vi "AB_850_860_Project_Source_Container.vi"(7 "action":T3, 8 "error in (no error)":errorcluster, 9 "index in":i32, 10 "dataSource in":T2, 11 "buildObject":T1) -> (0 "error out":errorcluster, 1 "index out":i32, 2 "dataSource out":T2, 3 "buildObject out":T1)   [LabVIEW 2020]
doc: "Reads and writes the data to the object property bag."
uses:
  <resource>/Framework/Providers/API/ItemRef.ctl
  <vilib>/AppBuilder/RW_Project/AB_RW_Project_PropBag_Action.ctl
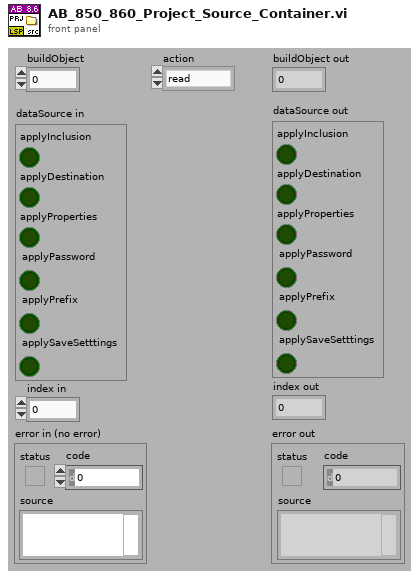
[diagram p1: front panel]
types:
  T1 = typedef "ItemRef.ctl" = u64
  T2 = cluster{"applyInclusion":bool, "applyDestination":bool, "applyProperties":bool, "applyPassword":bool, "applyPrefix":bool, "applySaveSetttings":bool}
  T3 = typedef "AB_RW_Project_PropBag_Action.ctl" = enum16{"read", "write", "clear", "readPrevious", "writePrevious", "clearPrevious"}
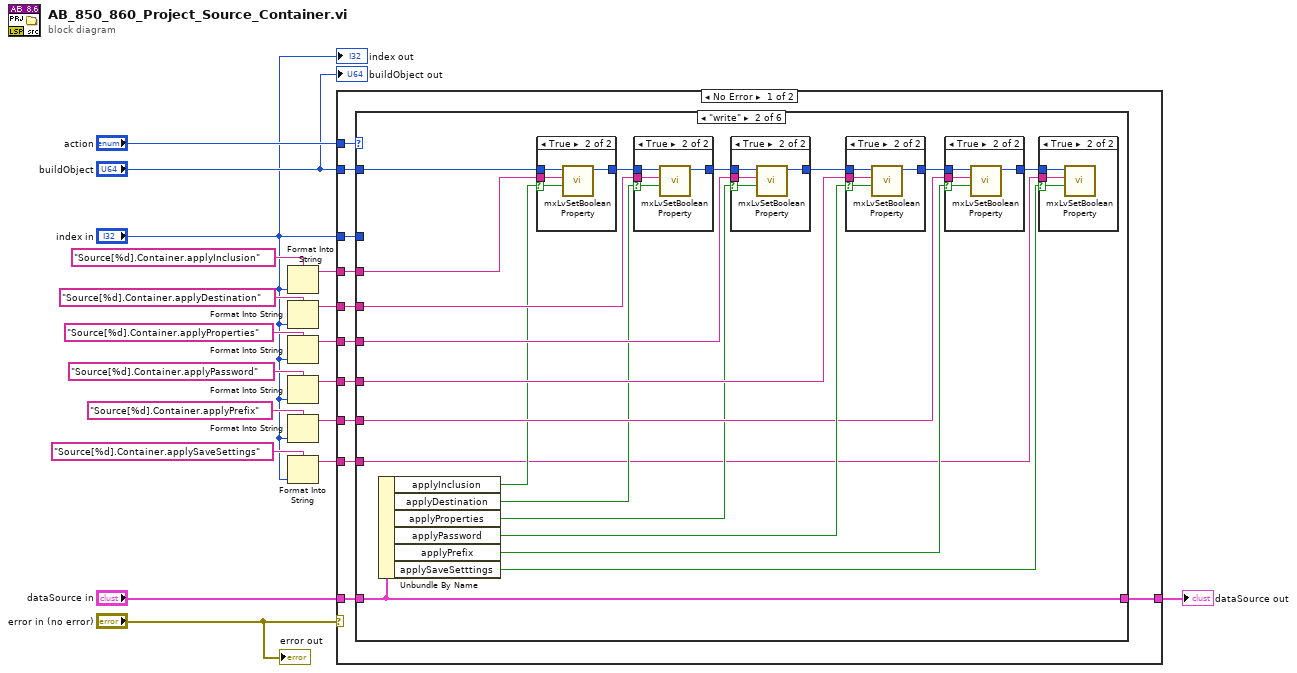
[diagram p0: block diagram]
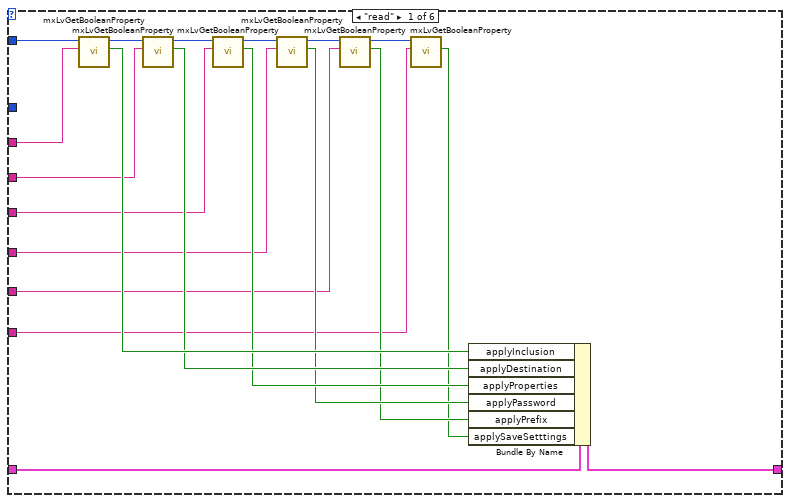
[diagram p2: hidden frame]
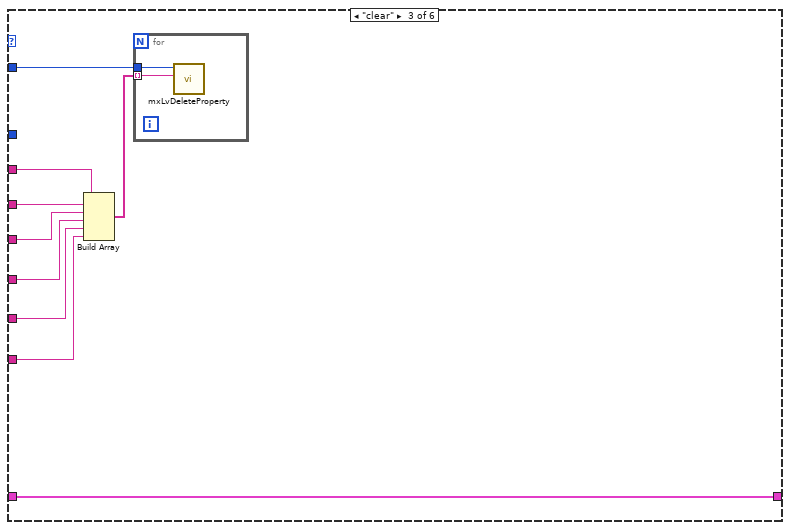
[diagram p9: hidden frame]
diagram:
  n1 = Format Into String(format string="Source[%d].Container.applyInclusion", "index in") -> (resulting string=w15:string)  [unwired: 2 in, 1 out]
  n2 = Format Into String(format string="Source[%d].Container.applyDestination", "index in") -> (resulting string=w12:string)  [unwired: 2 in, 1 out]
  n3 = Format Into String(format string="Source[%d].Container.applyProperties", "index in") -> (resulting string=w11:string)  [unwired: 2 in, 1 out]
  n4 = Format Into String(format string="Source[%d].Container.applyPassword", "index in") -> (resulting string=w6:string)  [unwired: 2 in, 1 out]
  n5 = Format Into String(format string="Source[%d].Container.applyPrefix", "index in") -> (resulting string=w4:string)  [unwired: 2 in, 1 out]
  n6 = Format Into String(format string="Source[%d].Container.applySaveSettings", "index in") -> (resulting string=w1:string)  [unwired: 2 in, 1 out]
  n7 = case shown="No Error" "error in (no error)" {
    tunnel: "action" -> [w29 _]
    tunnel: "dataSource in" -> [w28 w111]
    tunnel: w15 -> [w27 _]
    tunnel: w12 -> [w26 _]
    tunnel: w11 -> [w25 _]
    tunnel: "index in" -> [w24 _]
    tunnel: [w23 w111] -> w10
    tunnel: "buildObject" -> [w22 _]
    tunnel: w6 -> [w21 _]
    tunnel: w4 -> [w20 _]
    tunnel: w1 -> [w19 _]
    frame No Error {
      n8 = case shown="\"write\"" w29 {
        tunnel: w22 -> [w47 w65 w100 _ _ _]
        tunnel: w28 -> [w49 w68 w105 w108 w109 w110]
        tunnel: w27 -> [w45 w61 w104 _ _ _]
        tunnel: w26 -> [w42 w60 w103 _ _ _]
        tunnel: w25 -> [w40 w59 w102 _ _ _]
        tunnel: w24 -> [_ _ _ _ _ _]
        tunnel: [w48 w68 w105 w108 w109 w110] -> w23
        tunnel: w21 -> [w37 w67 w99 _ _ _]
        tunnel: w20 -> [w35 w57 w98 _ _ _]
        tunnel: w19 -> [w31 w51 w97 _ _ _]
        frame "read" {
          n9 = call <resource>:"mxLvGetBooleanProperty.vi"("Tag"=w45, "Item"=w47) -> ("Value"=w46:bool, "Item"=w44:T1)  [unwired: 1 in, 7 out]
          n10 = call <resource>:"mxLvGetBooleanProperty.vi"("Tag"=w42, "Item"=w44) -> ("Value"=w41:bool, "Item"=w43:T1)  [unwired: 1 in, 7 out]
          n11 = call <resource>:"mxLvGetBooleanProperty.vi"("Tag"=w40, "Item"=w43) -> ("Value"=w39:bool, "Item"=w38:T1)  [unwired: 1 in, 7 out]
          n12 = call <resource>:"mxLvGetBooleanProperty.vi"("Tag"=w37, "Item"=w38) -> ("Value"=w36:bool, "Item"=w34:T1)  [unwired: 1 in, 7 out]
          n13 = call <resource>:"mxLvGetBooleanProperty.vi"("Tag"=w35, "Item"=w34) -> ("Value"=w32:bool, "Item"=w33:T1)  [unwired: 1 in, 7 out]
          n14 = call <resource>:"mxLvGetBooleanProperty.vi"("Tag"=w31, "Item"=w33) -> ("Value"=w30:bool)  [unwired: 1 in, 8 out]
          n15 = Bundle By Name(cluster=w49, "applyInclusion"=w46, "applyDestination"=w41, "applyProperties"=w39, "applyPassword"=w36, "applyPrefix"=w32, "applySaveSetttings"=w30) -> (w48:T2)
        }
        frame "write" {
          n16 = Unbundle By Name(w68) -> ("applyInclusion"=w56:bool, "applyDestination"=w55:bool, "applyProperties"=w54:bool, "applyPassword"=w66:bool, "applyPrefix"=w53:bool, "applySaveSetttings"=w50:bool)
          n17 = case shown="True" w56 {
            selector: w56 -> [_ w89]
            tunnel: w65 -> [w87 w91]
            tunnel: w61 -> [_ w90]
            tunnel: [w87 w88] -> w64
            frame False {
            }
            frame True {
              n18 = call <resource>:"mxLvSetBooleanProperty.vi"("Value (F)"=w89, "Tag"=w90, "Item"=w91) -> ("Item"=w88:T1)  [unwired: 2 in, 6 out]
            }
          }
          n19 = case shown="True" w55 {
            selector: w55 -> [_ w84]
            tunnel: w64 -> [w82 w86]
            tunnel: w60 -> [_ w85]
            tunnel: [w82 w83] -> w58
            frame False {
            }
            frame True {
              n20 = call <resource>:"mxLvSetBooleanProperty.vi"("Value (F)"=w84, "Tag"=w85, "Item"=w86) -> ("Item"=w83:T1)  [unwired: 2 in, 6 out]
            }
          }
          n21 = case shown="True" w54 {
            selector: w54 -> [_ w79]
            tunnel: w58 -> [w77 w81]
            tunnel: w59 -> [_ w80]
            tunnel: [w77 w78] -> w63
            frame False {
            }
            frame True {
              n22 = call <resource>:"mxLvSetBooleanProperty.vi"("Value (F)"=w79, "Tag"=w80, "Item"=w81) -> ("Item"=w78:T1)  [unwired: 2 in, 6 out]
            }
          }
          n23 = case shown="True" w66 {
            selector: w66 -> [_ w94]
            tunnel: w63 -> [w92 w96]
            tunnel: w67 -> [_ w95]
            tunnel: [w92 w93] -> w62
            frame False {
            }
            frame True {
              n24 = call <resource>:"mxLvSetBooleanProperty.vi"("Value (F)"=w94, "Tag"=w95, "Item"=w96) -> ("Item"=w93:T1)  [unwired: 2 in, 6 out]
            }
          }
          n25 = case shown="True" w53 {
            selector: w53 -> [_ w74]
            tunnel: w62 -> [w72 w76]
            tunnel: w57 -> [_ w75]
            tunnel: [w72 w73] -> w52
            frame False {
            }
            frame True {
              n26 = call <resource>:"mxLvSetBooleanProperty.vi"("Value (F)"=w74, "Tag"=w75, "Item"=w76) -> ("Item"=w73:T1)  [unwired: 2 in, 6 out]
            }
          }
          n27 = case shown="True" w50 {
            selector: w50 -> [_ w69]
            tunnel: w52 -> [_ w71]
            tunnel: w51 -> [_ w70]
            frame False {
            }
            frame True {
              n28 = call <resource>:"mxLvSetBooleanProperty.vi"("Value (F)"=w69, "Tag"=w70, "Item"=w71) -> ()  [unwired: 2 in, 7 out]
            }
          }
        }
        frame "clear" {
          n29 = Build Array(w104, w103, w102, w99, w98, w97) -> (w101:string[])
          n30 = for {
            tunnel: w100 -> [w107]
            tunnel: w101 -> [w106] mode=indexing
            n31 = call <resource>:"mxLvDeleteProperty.vi"("Tag"=w106, "Item"=w107) -> ()  [unwired: 1 in, 9 out]
          }
        }
        frame "readPrevious" {
        }
        frame "writePrevious" {
        }
        frame "clearPrevious" {
        }
      }
    }
    frame Error {
    }
  }
  "dataSource out" <- w10
  "error out" <- "error in (no error)"
  "buildObject out" <- "buildObject"
  "index out" <- "index in"
